vi "test Get Attribute as JSON Multiple Sheets.vi"(11 "Test Case In":refnum<class "Test Config From Excel Table.lvclass">) -> (0 "error out":errorcluster, 3 "Test Case Out":refnum<class "Test Config From Excel Table.lvclass">)   [LabVIEW 2020, in "Test Config From Excel Table.lvclass"]
uses:
  Test Config From Excel Table.lvclass
  C:/Program Files/National Instruments/LabVIEW 2025/vi.lib/Astemes/LUnit/Test Case.lvclass
  Source/Config from Excel Table/Config from Excel Table.lvclass
  <vilib>/Astemes/LUnit/Test Case.lvclass/Test Case.ctl
  <vilib>/JDP Science/JSONtext/JSONtext.lvlib
  <vilib>/Astemes/LUnit/Test Case.lvclass
  <vilib>/Peter/Open Xml/Source/Open Xml.lvlib
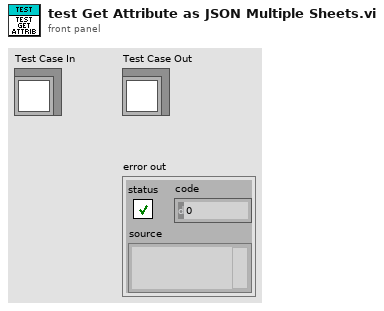
[diagram p1: front panel]
types:
  T1 = cluster{"Sheet Name":string, "Name":string, "Display Name":string, "Range or Cell Address":string}
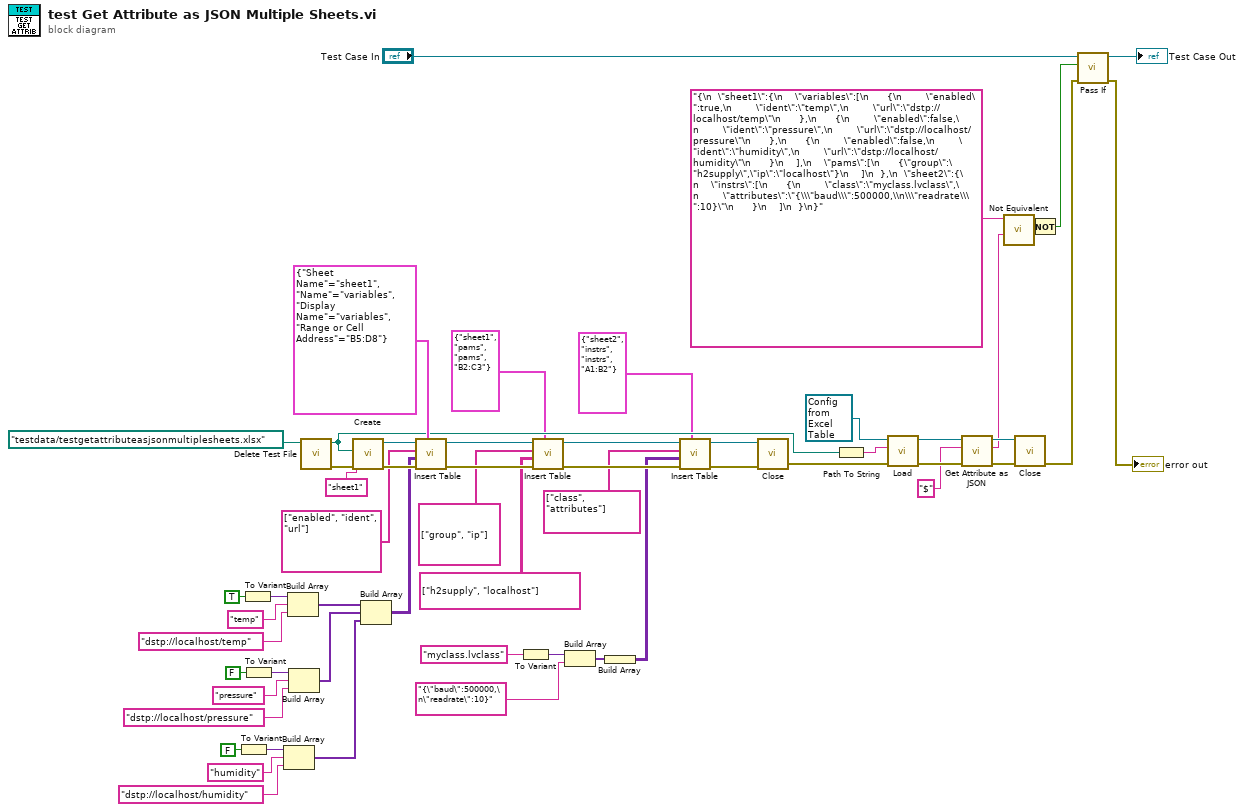
[diagram p0: block diagram]
diagram:
  n1 = To Variant(anything=FALSE) -> (Variant=w30:variant)
  n2 = To Variant(anything=TRUE) -> (Variant=w39:variant)
  n3 = To Variant(anything=FALSE) -> (Variant=w33:variant)
  n4 = Build Array(w30, "humidity", "dstp://localhost/humidity") -> (w26:variant[])
  n5 = Build Array(w39, "temp", "dstp://localhost/temp") -> (w36:variant[])
  n6 = Build Array(w33, "pressure", "dstp://localhost/pressure") -> (w27:variant[])
  n7 = call "Delete Test File.vi"("name or relative path"=path "testdata/testgetattributeasjsonmultiplesheets.xlsx") -> ("error out"=w44:errorcluster, "deleted path"=w19:path)  [unwired: 9 in]
  n8 = call <vilib>:"Create.vi"("error in"=w44, "SheetName"="sheet1", "Path"=w19) -> ("error out"=w43:errorcluster, "SpreadsheetDoc"=w24:refnum<k24>)  [unwired: 7 in]
  n9 = Build Array(w36, w27, w26) -> (w25:variant[][])
  n10 = call <vilib>:"Insert Table.vi"("Location"=T1 {"Sheet Name"="sheet1", "Name"="variables", "Display Name"="variables", "Range or Cell Address"="B5:D8"}, "error in"=w43, "Cell Values"=w25, "Header Names"=string[] ["enabled", "ident", "url"], "SpreadsheetDoc in"=w24) -> ("error out"=w23:errorcluster, "SpreadsheetDoc out"=w16:refnum<k24>)  [unwired: 5 in]
  n11 = To Variant(anything="myclass.lvclass") -> (Variant=w2:variant)
  n12 = call <vilib>:"Insert Table.vi"("Location"=T1 {"Sheet Name"="sheet1", "Name"="pams", "Display Name"="pams", "Range or Cell Address"="B2:C3"}, "error in"=w23, "Cell Values"=string[][] [["h2supply", "localhost"]] ("Header Names"), "Header Names"=string[] ["group", "ip"], "SpreadsheetDoc in"=w16) -> ("error out"=w17:errorcluster, "SpreadsheetDoc out"=w10:refnum<k24>)  [unwired: 5 in]
  n13 = Build Array(w2, "{\"baud\":500000,\n\"readrate\":10}" ("element")) -> (w4:variant[])
  n14 = Build Array(w4) -> (w3:variant[][])
  n15 = call <vilib>:"Insert Table.vi"("Location"=T1 {"Sheet Name"="sheet2", "Name"="instrs", "Display Name"="instrs", "Range or Cell Address"="A1:B2"}, "error in"=w17, "Cell Values"=w3, "Header Names"=string[] ["class", "attributes"], "SpreadsheetDoc in"=w10) -> ("error out"=w11:errorcluster, "SpreadsheetDoc out"=w9:refnum<k24>)  [unwired: 5 in]
  n16 = call <vilib>:"Close.vi"("error in"=w11, "SpreadsheetDoc"=w9) -> ("error out"=w22:errorcluster)  [unwired: 9 in]
  n17 = Path To String(path=w19) -> (string=w53:string)
  n18 = call-dynamic "Load.vi"("error in"=w22, "Source"=w53, "Config from Excel Table in"=refnum<class "Config from Excel Table.lvclass"> refnum ("Config from EXCEL Table.lvclass")) -> ("error out"=w50:errorcluster, "Config from Excel Table out"=w51:refnum<class "Config from Excel Table.lvclass">)  [unwired: 7 in]
  n19 = call-dynamic "Get Attribute as JSON.vi"("error in"=w50, "Attribute"="$", "Config from Excel Table in"=w51) -> ("error out"=w48:errorcluster, "<JSON>"=w18:string, "Config from Excel Table out"=w47:refnum<class "Config from Excel Table.lvclass">)  [unwired: 6 in]
  n20 = call <vilib>:"Not Equivalent.vi"("Other JSON"=w18, "JSON"="{\n  \"sheet1\":{\n    \"variables\":[\n      {\n        \"enabled\":true,\n        \"ident\":\"temp\",\n        \"url\":\"dstp://localhost/temp\"\n      },\n      {\n        \"enabled\":false,\n        \"ident\":\"pressure\",\n        \"url\":\"dstp://localhost/pressure\"\n      },\n      {\n        \"enabled\":false,\n        \"ident\":\"humidity\",\n        \"url\":\"dstp://localhost/humidity\"\n      }\n    ],\n    \"pams\":[\n      {\"group\":\"h2supply\",\"ip\":\"localhost\"}\n    ]\n  },\n  \"sheet2\":{\n    \"instrs\":[\n      {\n        \"class\":\"myclass.lvclass\",\n        \"attributes\":\"{\\\"baud\\\":500000,\\n\\\"readrate\\\":10}\"\n      }\n    ]\n  }\n}") -> ("Not Equivalent"=w46:bool)  [unwired: 8 in]
  n21 = call-dynamic <vilib>:"Close.vi"("error in"=w48, "Config from Excel Table in"=w47) -> ("error out"=w52:errorcluster)  [unwired: 8 in, 1 out]
  n22 = Not(x=w46) -> (.not. x?=w45:bool)
  n23 = call <vilib>:"Pass If.vi"("error in (no error)"=w52, "Pass?"=w45, "LUnit Test Case In"="Test Case In") -> ("error out"=→"error out":errorcluster, "LUnit Test Case Out"=→"Test Case Out":refnum<class "Test Config From Excel Table.lvclass">)  [unwired: 7 in]
